vi "RF_RxParaConf.vi"(8 "error in":errorcluster, 10 "DeviceConfiguare":T2, 11 "VISA IN":T1={"端口选择"=" ", "波特率"=115200, "数据位"=8, "奇偶校验"=0, "停止位"=10, "流控"=0} {"流控" items=["None"=0, "XON/XOFF"=1, "RTS/CTS"=2, "DTR/DSR"=4]; "停止位" items=["1.0"=10, "1.5"=15, "2.0"=20]; "奇偶校验" items=["None", "Odd", "Even", "Mark", "Space"]; "数据位" min=5 max=8 step=1}) -> (0 "error out":errorcluster, 3 "VISA OUT":T1={"端口选择"=" ", "波特率"=115200, "数据位"=8, "奇偶校验"=0, "停止位"=10, "流控"=0} {"流控" items=["None"=0, "XON/XOFF"=1, "RTS/CTS"=2, "DTR/DSR"=4]; "停止位" items=["1.0"=10, "1.5"=15, "2.0"=20]; "奇偶校验" items=["None", "Odd", "Even", "Mark", "Space"]; "数据位" min=5 max=8 step=1})   [LabVIEW 2015]
uses:
  <vilib>/Instr/_visa.llb/VISA Flush IO Buffer Mask.ctl
  <vilib>/Instr/_visa.llb/VISA Configure Serial Port (Instr).vi
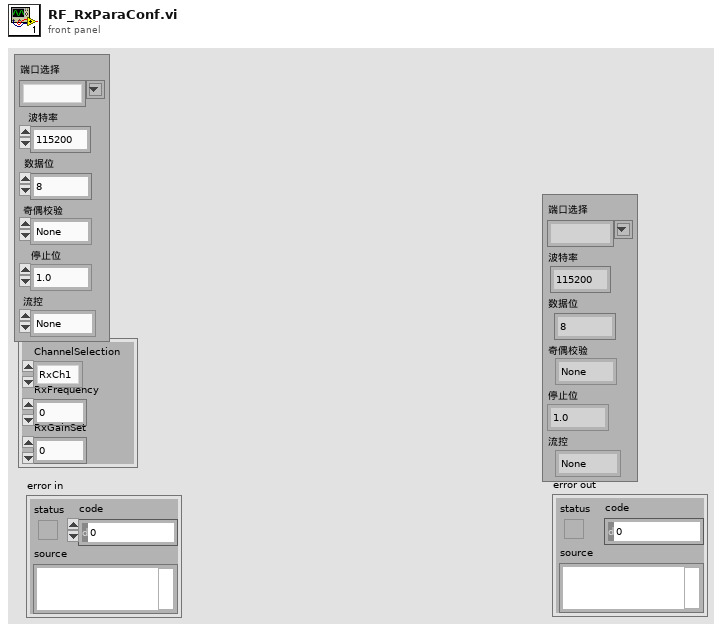
[diagram p1: front panel]
types:
  T1 = cluster{"端口选择":string, "波特率":u32, "数据位":u16, "奇偶校验":u16, "停止位":u16, "流控":u16}
  T2 = cluster{"ChannelSelection":enum16{"RxCh1", "RxCh2"}, "RxFrequency":u32, "RxGainSet":u8}
  T3 = typedef "VISA Flush IO Buffer Mask.ctl" = u16
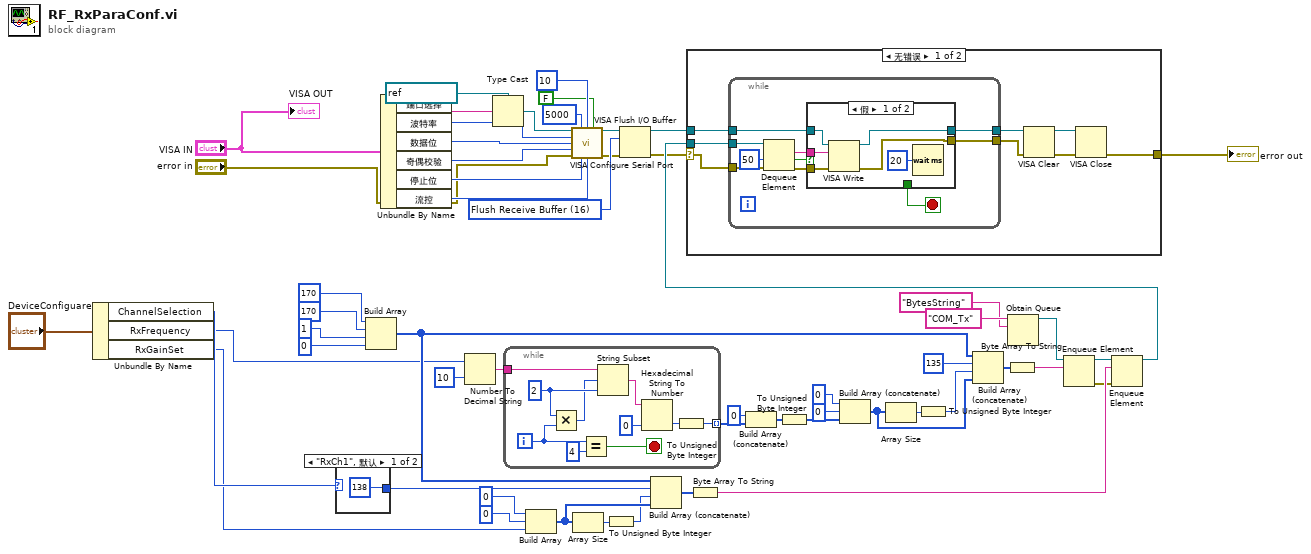
[diagram p0: block diagram]
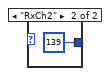
[diagram p2: hidden frame]
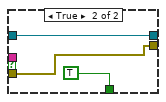
[diagram p3: hidden frame]
diagram:
  w13 = T3 16 items=["Flush Receive Buffer"=16, "Write Transmit Buffer to Device"=32, "Flush Receive Buffer (No I/O)"=64, "Flush Transmit Buffer"=128] ("Mask")
  n1 = Unbundle By Name("DeviceConfiguare") -> ("ChannelSelection"=w50:enum16{"RxCh1", "RxCh2"}, "RxFrequency"=w26:u32, "RxGainSet"=w42:u8)
  n2 = case shown="\"RxCh1\", 默认" w50 {
    tunnel: [u8 138 u8 139] -> w49
    frame "RxCh1", Default {
    }
    frame "RxCh2" {
    }
  }
  n3 = Build Array(u8 170, u8 170, u8 1, u8 0) -> (w41:u8[])
  n4 = Unbundle By Name("VISA IN") -> ("端口选择"=w15:string, "波特率"=w9:u32, "数据位"=w5:u16, "奇偶校验"=w6:u16, "停止位"=w7:u16, "流控"=w8:u16)
  n5 = Number To Decimal String(number=w26, width (-)=i16 10 ("宽度(-)")) -> (decimal integer string=w40:string)
  n6 = Type Cast(type=refnum<visa-resource-name> "COM15" ("VISA resource name"), x=w15) -> (*(type *) &x=w17:refnum<visa-resource-name>)
  n7 = while {
    tunnel: w40 -> [w66]
    tunnel: [w59] -> w24 mode=indexing
    i -> [w64]
    stop <- w67 stop-if-true
    w65 = 2 ("长度（剩余）")
    n8 = Multiply(x=w65, y=w64) -> (x*y=w63:i32)
    n9 = Equal?(x=w64, y=4) -> (x = y?=w67:bool)
    n10 = String Subset(string=w66, offset (0)=w63, length (rest)=w65) -> (substring=w61:string)
    n11 = Hexadecimal String To Number(string=w61, default (0uL)=u8 0 ("默认(0 U32)")) -> (number=w60:u8)  [unwired: 2 out]
    n12 = To Unsigned Byte Integer(number=w60) -> (unsigned 8bit integer=w59:u8)
  }
  n13 = Build Array(u8 0, u8 0, w42) -> (w47:u8[])
  n14 = call-poly "VISA Configure Serial Port"("VISA resource name"=w17, "timeout (10sec)"=u32 5000, "termination char\n(0xA = '\\n' = LF)"=u8 10 ("termination char\n(0xA = '\\n' = LF)"), "Enable Termination\nChar (T)"=FALSE ("Enable Termination Char (T)"), "baud rate (9600)"=w9, "data bits (8)"=w5, "parity (0:none)"=w6, "error in (no error)"="error in", "stop bits (10: 1 bit)"=w7, "flow control (0:none)"=w8) -> ("VISA resource name out"=w11:refnum<visa-resource-name>, "error out"=w12:errorcluster)  [unwired: 4 out]
  n15 = Array Size(array=w47) -> (size(s)=w45:i32)
  n16 = To Unsigned Byte Integer(number=w45) -> (unsigned 8bit integer=w46:u8)
  n17 = VISA Flush I/O Buffer(VISA resource name=w11, mask (16)=w13, error in (no error)=w12) -> (VISA resource name out=w21:refnum<visa-resource-name>, error out=w20:errorcluster)
  n18 = Build Array (concatenate)(w41, w49, w46, w47) -> (w48:u8[])
  n19 = Byte Array To String(unsigned byte array=w48) -> (string=w55:string)
  n20 = Build Array (concatenate)(u8 0 ("射频类型"), w24) -> (w25:u8[])
  n21 = To Unsigned Byte Integer(number=w25) -> (unsigned 8bit integer=w28:u8[])
  n22 = Build Array (concatenate)(u8 0, u8 0, w28) -> (w37:u8[])
  n23 = Array Size(array=w37) -> (size(s)=w35:i32)
  n24 = To Unsigned Byte Integer(number=w35) -> (unsigned 8bit integer=w36:u8)
  n25 = Build Array (concatenate)(w41, u8 135, w36, w37) -> (w38:u8[])
  n26 = Byte Array To String(unsigned byte array=w38) -> (string=w52:string)
  n27 = Obtain Queue(name (unnamed)="COM_Tx", element data type="BytesString" ("name (unnamed)")) -> (queue out=w51:refnum<queue>)  [unwired: 3 in, 2 out]
  n28 = Enqueue Element(queue=w51, element=w52) -> (queue out=w53:refnum<queue>, error out=w54:errorcluster)  [unwired: 1 in, 2 out]
  n29 = Enqueue Element(queue=w53, element=w55, error in (no error)=w54) -> (queue out=w56:refnum<queue>)  [unwired: 3 out]
  n30 = case shown="无错误" w20 {
    selector: w20 -> [w70 w96]
    tunnel: w56 -> [w76 _]
    tunnel: w21 -> [w75 _]
    tunnel: [w71 w96] -> w3
    frame No Error {
      n31 = while {
        tunnel: w76 -> [w86]
        tunnel: w75 -> [w81]
        tunnel: [w79] -> w74
        tunnel: w70 -> [w78]
        tunnel: [w77] -> w69
        stop <- w80 stop-if-true
        n32 = Dequeue Element(queue=w86, timeout in ms (-1)=50, error in (no error)=w78) -> (element=w82:string, timed out?=w83:bool, error out=w84:errorcluster)  [unwired: 1 out]
        n33 = case shown="假" w83 {
          tunnel: w84 -> [w92 w93]
          tunnel: w82 -> [w91 _]
          tunnel: w81 -> [w89 w94]
          tunnel: [_ TRUE] -> w80
          tunnel: [w88 w94] -> w79
          tunnel: [w87 w93] -> w77
          frame False {
            n34 = VISA Write(VISA resource name=w89, write buffer=w91, error in (no error)=w92) -> (VISA resource name out=w88:refnum<visa-resource-name>, error out=w87:errorcluster)  [unwired: 1 out]
            n35 = Wait (ms)(milliseconds to wait=u32 20) -> ()  [unwired: 1 out]
          }
          frame True {
          }
        }
      }
      n36 = VISA Clear(VISA resource name=w74, error in (no error)=w69) -> (VISA resource name out=w73:refnum<visa-resource-name>, error out=w72:errorcluster)
      n37 = VISA Close(VISA resource name=w73, error in (no error)=w72) -> (error out=w71:errorcluster)
    }
    frame Error {
    }
  }
  "error out" <- w3
  "VISA OUT" <- "VISA IN"
